vi "Read Axes.vi"(8 "error in (no error)":errorcluster, 11 "Focus Class in":refnum<class "Focus Class.lvclass">) -> (0 "error out":errorcluster, 2 "Axes":i32=3, 3 "Focus Class out":refnum<class "Focus Class.lvclass">)   [LabVIEW 2022 SP3, in "Focus Class.lvclass"]
uses:
  Focus Class.lvclass
  Focus Class.lvclass/Focus Class.ctl
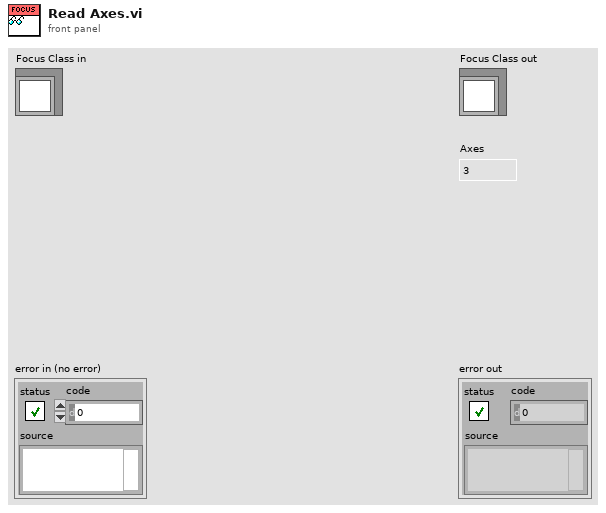
[diagram p1: front panel]
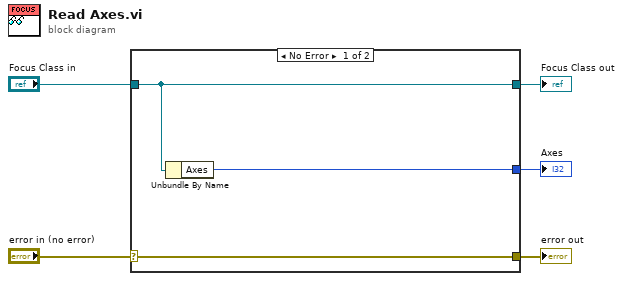
[diagram p0: block diagram]
diagram:
  n1 = case shown="No Error" "error in (no error)" {
    selector: "error in (no error)" -> [w8 w9]
    tunnel: [w8 w9] -> w4
    tunnel: [w7 w10] -> w2
    tunnel: "Focus Class in" -> [w7 w10]
    tunnel: [w6 _] -> w1
    frame No Error {
      n2 = Unbundle By Name(w7) -> ("Axes"=w6:i32)
    }
    frame Error {
    }
  }
  "error out" <- w4
  "Focus Class out" <- w2
  "Axes" <- w1
